vi "Polar to Cartesian.vi"(8 "Phi":dbl, 11 "B":dbl) -> (0 "Y":dbl, 3 "Z":dbl)   [LabVIEW 2019]
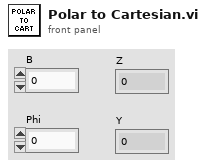
[diagram p1: front panel]
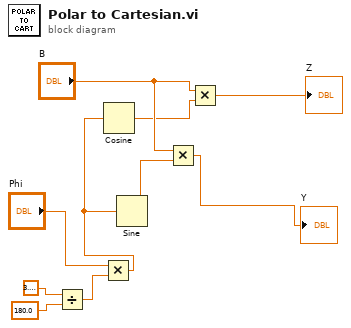
[diagram p0: block diagram]
diagram:
  n1 = Divide(x=3.141592653589793, y=180.0) -> (x/y=w2:dbl)
  n2 = Multiply(x="Phi", y=w2) -> (x*y=w1:dbl)
  n3 = Cosine(x=w1) -> (cos(x)=w6:dbl)
  n4 = Sine(x=w1) -> (sin(x)=w10:dbl)
  n5 = Multiply(x="B", y=w10) -> (x*y=→"Y":dbl)
  n6 = Multiply(x="B", y=w6) -> (x*y=→"Z":dbl)
